vi "get_radar_config_params.vi"(4 "error in":errorcluster, 7 "Radar configuration":string="{\n  \"type\": \"Radar\",\n   \"gpu_number\":0,\n  \"listen_port\": 8301,\n  \"send_radar_cube\":false,\n  \"paint_targets\": false,\n  \"target_paint_lifetime\": 0.5,\n  \"location\": {\n    \"x\": 250.0,\n    \"y\": 0.0,\n    \"z\": 50.0\n  },\n  \"rotation\": {\n    \"pitch\": 0.0,\n    \"yaw\": 0.0,\n    \"roll\": 0.0\n  },\n  \"num_samples_per_sweep\":345,\n  \"fs\": 50000000,\n  \"fc\": 77000000000.0,\n  \"num_sweeps\": 32,\n  \"sweep_time\" : 0.0000069,\n  \"bandwidth\" : 172500000,\n  \"max_targets\": 250,\n  \"elements\": 8,\n  \"transmitter\": {\n    \"peak_power\": 5.0,\n    \"aperture\": 0.000859,\n    \"gain\": 13.50\n  },\n  \"receiver\": {\n    \"aperture\": 0.000798,\n    \"nf\": 10.0,\n    \"noise_temp\": 290.0,\n    \"nb\": 74000000.0,\n    \"gain\": 10.0\n  },\n  \"sbr\": {\n    \"long_range_scan_distance\": 150.0,\n    \"short_range_scan_distance\": 60.0,\n    \"long_range_fov\": 20.0,\n    \"short_range_fov\": 60.0,\n    \"elevation_fov\": 10.0,\n    \"rescan_density\": 20.0,\n    \"debug_frustum\": false,\n    \"debug_scan\": false,\n    \"debug_rescan\": false\n  }\n}") -> (0 "error out":errorcluster, 1 "num_samples_per_sweep":dbl, 2 "num_sweeps":dbl, 3 "elements":dbl)   [LabVIEW 2019, in "Lib_Simx.lvlib"]
doc: "Parses the configuration an obtain the following parameters: elements, the number of sweeps and number of samples per sweep."
uses:
  Lib_Simx.lvlib
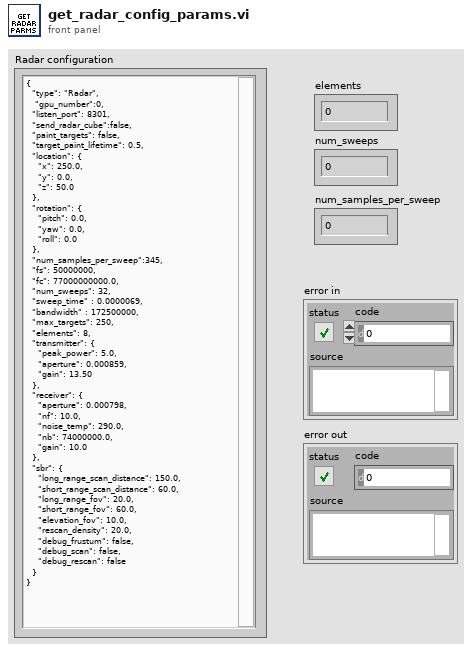
[diagram p1: front panel]
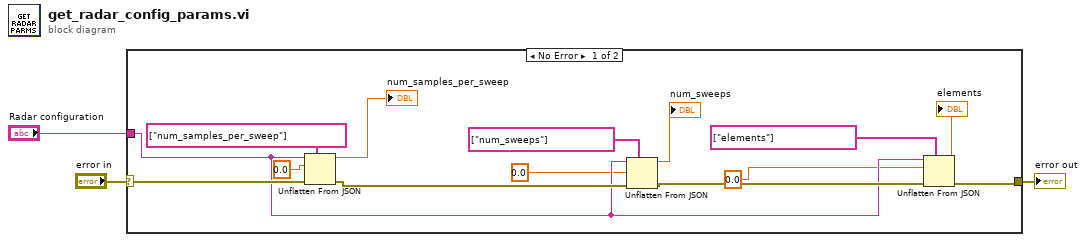
[diagram p0: block diagram]
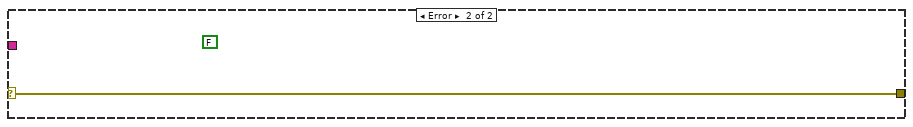
[diagram p2: hidden frame]
diagram:
  n1 = case shown="No Error" "error in" {
    selector: "error in" -> [w15 w18]
    tunnel: "Radar configuration" -> [w10 _]
    tunnel: [w9 w18] -> w2
    frame No Error {
      n2 = Unflatten From JSON(path=string[] ["num_samples_per_sweep"], JSON string=w10, type and defaults=0.0, error in (no error)=w15) -> (value=→"num_samples_per_sweep":dbl, error out=w12:errorcluster)  [unwired: 3 in]
      n3 = Unflatten From JSON(path=string[] ["num_sweeps"], JSON string=w10, type and defaults=0.0, error in (no error)=w12) -> (value=→"num_sweeps":dbl, error out=w11:errorcluster)  [unwired: 3 in]
      n4 = Unflatten From JSON(path=string[] ["elements"], JSON string=w10, type and defaults=0.0, error in (no error)=w11) -> (value=→"elements":dbl, error out=w9:errorcluster)  [unwired: 3 in]
    }
    frame Error {
      (unwired) FALSE ("f")
    }
  }
  "error out" <- w2
